vi "SpreadsheetRead.vi"() -> (2 "output cluster":cluster{"X Array":dbl[], "Y Array":dbl[]})   [LabVIEW 2014]
uses:
  <vilib>/Utility/file.llb/Read From Spreadsheet File (DBL).vi
panel:
  out "XY Graph":cluster{"all rows":dbl[], "all rows":dbl[]}(graph)
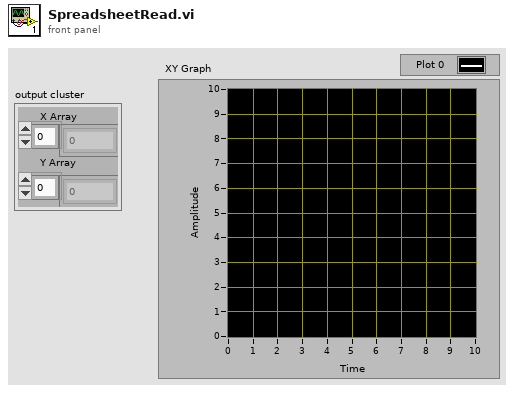
[diagram p1: front panel]
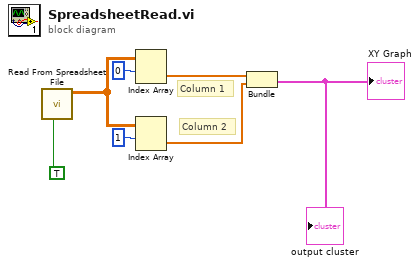
[diagram p0: block diagram]
diagram:
  # "Column 2"
  # "Column 1"
  n1 = call-poly <vilib>:"Read From Spreadsheet File.vi"("transpose (no:F)"=TRUE) -> ("all rows"=w7:dbl[][])  [unwired: 6 in, 4 out]
  n2 = Index Array(array=w7, index (row)=0) -> (element=w4:dbl[])  [unwired: 1 in]
  n3 = Index Array(array=w7, index (row)=1) -> (element=w3:dbl[])  [unwired: 1 in]
  n4 = Bundle("all rows"=w4, "all rows"=w3) -> (→"XY Graph" →"output cluster":cluster{"all rows":dbl[], "all rows":dbl[]})  [unwired: 1 in]
